vi "init.vi"(8 "error in (no error)":errorcluster, 10 "WeatherData":refnum<class "WeatherData.lvclass">, 11 "DisplayBase in":refnum<class "DisplayBase.lvclass">) -> (0 "error out":errorcluster, 3 "DisplayBase out":refnum<class "DisplayBase.lvclass">)   [LabVIEW 2020, in "DisplayBase.lvclass"]
uses:
  DisplayBase.lvclass
  C:/Projects/Repos/HeadFirstDesignPatterns/HeadFirstDesignPatternsLabVIEWandPython/02 Observer/LabVIEW/Observer/Observer.lvclass
  WeatherData/WeatherData.lvclass
  DisplayBase.lvclass/DisplayBase.ctl
panel:
  # "Connector Pane"
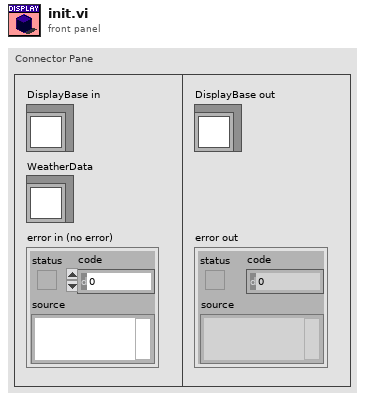
[diagram p1: front panel]
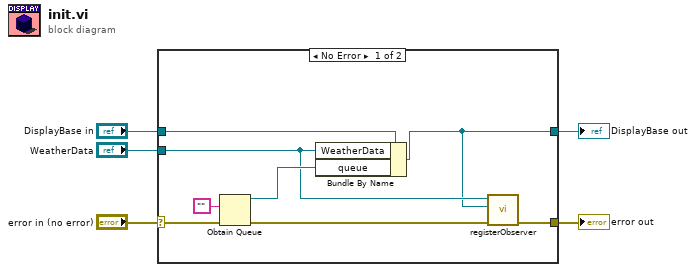
[diagram p0: block diagram]
diagram:
  n1 = case shown="No Error" "error in (no error)" {
    selector: "error in (no error)" -> [w12 w14]
    tunnel: [w8 w14] -> w4
    tunnel: [w6 w15] -> w2
    tunnel: "DisplayBase in" -> [w11 w15]
    tunnel: "WeatherData" -> [w7 _]
    frame No Error {
      n2 = Obtain Queue(element data type="", error in (no error)=w12) -> (queue out=w13:refnum<queue>, error out=w9:errorcluster)  [unwired: 3 in, 1 out]
      n3 = Bundle By Name(cluster=w11, "WeatherData"=w7, "queue"=w13) -> (w6:refnum<class "DisplayBase.lvclass">)
      n4 = call-dynamic "registerObserver.vi"("error in (no error)"=w9, "Observer.lvclass"=w6, "WeatherData.lvclass"=w7) -> ("error out"=w8:errorcluster)  [unwired: 7 in, 1 out]
    }
    frame Error {
    }
  }
  "error out" <- w4
  "DisplayBase out" <- w2
